vi "NOT16.vi"(1 "A":bool[](array[boolean])=[FALSE, FALSE, FALSE, FALSE, FALSE, FALSE, FALSE, FALSE, FALSE, FALSE, FALSE, FALSE, FALSE, FALSE, FALSE, FALSE]) -> (0 "z":bool[](array[boolean]))   [LabVIEW 2012]
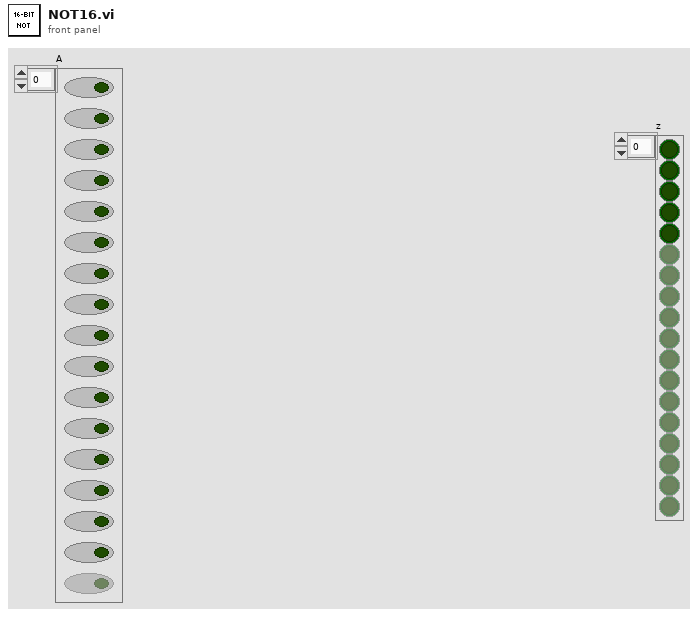
[diagram p1: front panel]
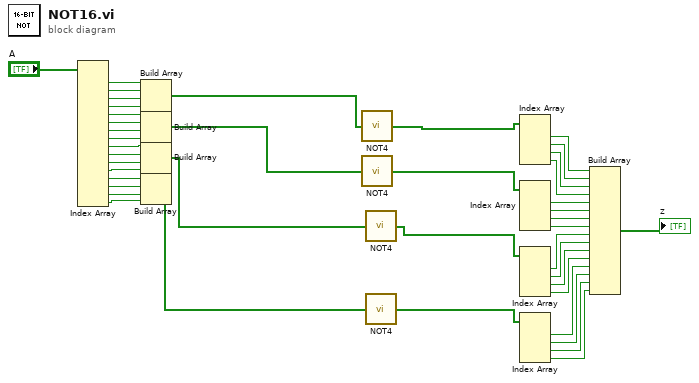
[diagram p0: block diagram]
diagram:
  n1 = Index Array(array="A") -> (element #1=w42:bool, element #2=w41:bool, element #3=w40:bool, element #4=w39:bool, element #5=w38:bool, element #6=w37:bool, element #7=w36:bool, element #8=w35:bool, element #9=w34:bool, element #10=w33:bool, element #11=w32:bool, element #12=w31:bool, element #13=w30:bool, element #14=w29:bool, element #15=w28:bool, element #16=w27:bool)  [unwired: 16 in]
  n2 = Build Array(w42, w41, w40, w39) -> (w4:bool[])
  n3 = Build Array(w38, w37, w36, w35) -> (w3:bool[])
  n4 = Build Array(w34, w33, w32, w31) -> (w2:bool[])
  n5 = Build Array(w30, w29, w28, w27) -> (w1:bool[])
  n6 = call "NOT4.vi"("A"=w4) -> ("z"=w8:bool[])
  n7 = call "NOT4.vi"("A"=w3) -> ("z"=w7:bool[])
  n8 = call "NOT4.vi"("A"=w2) -> ("z"=w6:bool[])
  n9 = call "NOT4.vi"("A"=w1) -> ("z"=w5:bool[])
  n10 = Index Array(array=w8) -> (element #1=w26:bool, element #2=w25:bool, element #3=w24:bool, element #4=w23:bool)  [unwired: 4 in]
  n11 = Index Array(array=w7) -> (element #1=w22:bool, element #2=w21:bool, element #3=w20:bool, element #4=w19:bool)  [unwired: 4 in]
  n12 = Index Array(array=w6) -> (element #1=w18:bool, element #2=w17:bool, element #3=w16:bool, element #4=w15:bool)  [unwired: 4 in]
  n13 = Index Array(array=w5) -> (element #1=w14:bool, element #2=w13:bool, element #3=w12:bool, element #4=w11:bool)  [unwired: 4 in]
  n14 = Build Array(w26, w25, w24, w23, w22, w21, w20, w19, w18, w17, w16, w15, w14, w13, w12, w11) -> (→"z":bool[])
